vi "Framework Page.vi"(8 "error in (no error)":errorcluster, 11 "Node Ptr":T1 format="%.0x") -> (0 "error out":errorcluster)   [LabVIEW 2019, in "DSF System Explorer.lvlib"]
uses:
  DSF System Explorer.lvlib
  <vilib>/NI VeriStand/Custom Device API/Custom Device API.lvlib
  Shared/DSF Shared.lvlib
  <vilib>/NI VeriStand/Custom Device API/Custom Device Item Ref.ctl
panel:
  in  "SHDocVw.IWebBrowser":refnum<k7>(container)
  in  "New":bool
  in  "Configuration Version":string
  in  "Export":bool
  in  "Debug Mode":bool
  in  "Launch Data Viewer":bool
  in  "Server Frequency":dbl(ring)=20.0 items=["0.5 Hz"=0.5, "1.0 Hz"=1.0, "2.0 Hz"=2.0, "2.5 Hz"=2.5, "4.0 Hz"=4.0, "5.0 Hz"=5.0, "8.0 Hz"=8.0, "10.0 Hz"=10.0, "12.5 Hz"=12.5, "20.0 Hz"=20.0, "25.0 Hz"=25.0, "40.0 Hz"=40.0, "50.0 Hz"=50.0, "100.0 Hz"=100.0]
  in  "Enable Data Server":bool
  in  "Show Dialog on Error":bool
  in  "Show Threads":bool
  in  "Infinite FIFO Timeouts":bool
  in  "Measure Durations":bool
  in  "Measure Period":bool
  in  "Import":bool
  in  "View Configuration":bool
  # "Debug Options"
  # "Measurement Options"
  # "Data Server Options"
  # "All Targets"
  # "All Targets"
  # "All Targets"
  # "Windows Only"
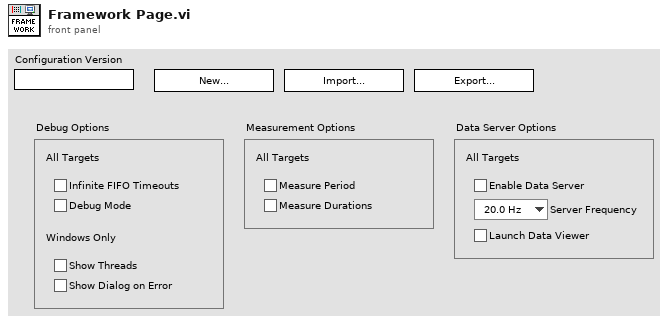
[diagram p1: front panel]
types:
  T1 = typedef "Custom Device API.lvlib/Custom Device Item Ref.ctl" = u64
  T2 = typedef "DSF Core.lvlibp/Framework.lvclass/Framework Options.ctl" = cluster{"FIFO Options":T3, "Thread Options":T4, "Plugin Options":T5, "Performance Options":T6, "Data Server Options":T7}
  T3 = typedef "DSF Core.lvlibp/Framework.lvclass/DSF FIFO Options.ctl" = cluster{"Infinite Timeouts":bool}
  T4 = typedef "DSF Core.lvlibp/Thread.lvclass/Thread Options.ctl" = cluster{"Show FP On Call":bool, "Close FP After Call":bool, "Allow Debugging":bool}
  T5 = typedef "DSF Core.lvlibp/Framework.lvclass/DSF Plugin Options.ctl" = cluster{"Default Components":bool}
  T6 = typedef "DSF Core.lvlibp/DSF Performance Options.ctl" = cluster{"Measure Period":bool, "Measure Rx/Tx Duration":bool}
  T7 = typedef "DSF Core.lvlibp/Framework.lvclass/Data Server Options.ctl" = cluster{"Enable Data Server":bool, "Period":u32}
  T8 = typedef "DSF Core.lvlibp/DSF Version Info.ctl" = cluster{"major":u32, "minor":u32, "fix":u32, "build":string}
  T9 = typedef "Custom Device API.lvlib/Custom Device Commands.ctl" = enum16{"Default", "Item renamed", "Shutdown", "Dynamic button pressed"}
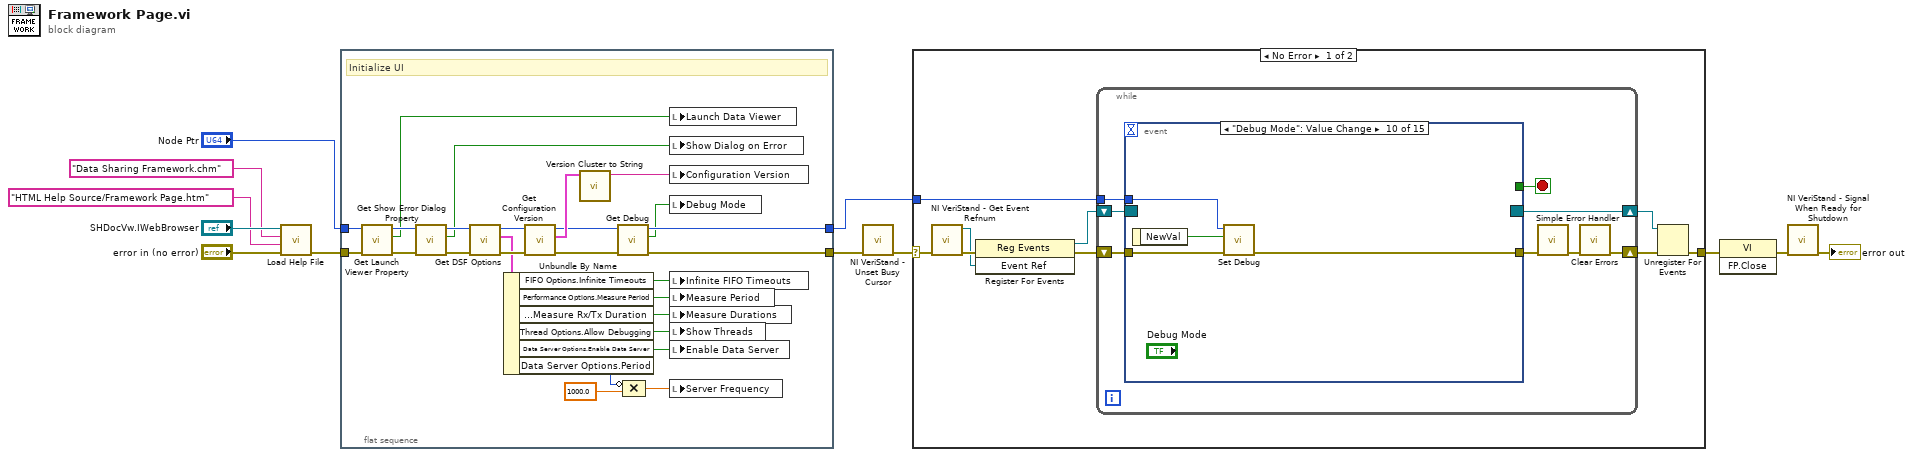
[diagram p0: block diagram]
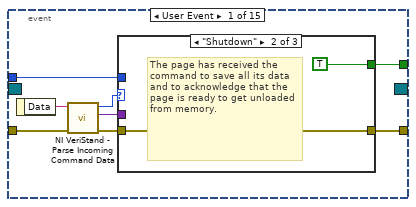
[diagram p2: hidden frame]
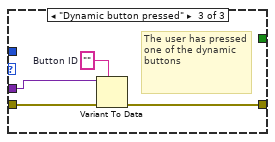
[diagram p4: hidden frame]
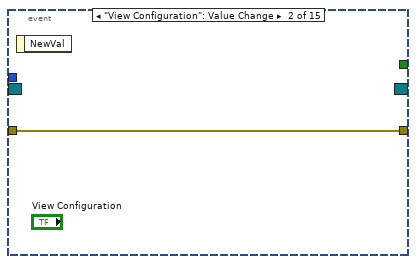
[diagram p5: hidden frame]
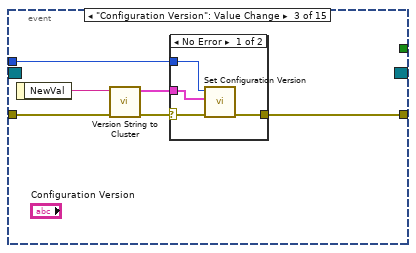
[diagram p6: hidden frame]
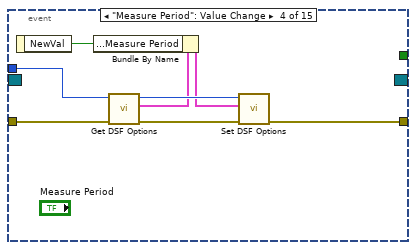
[diagram p8: hidden frame]
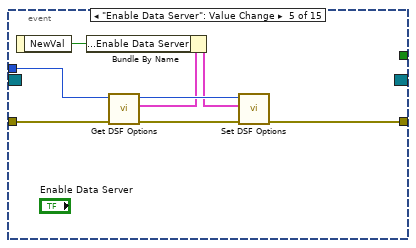
[diagram p9: hidden frame]
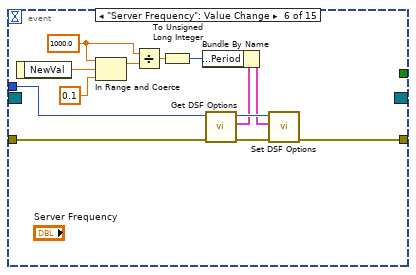
[diagram p10: hidden frame]
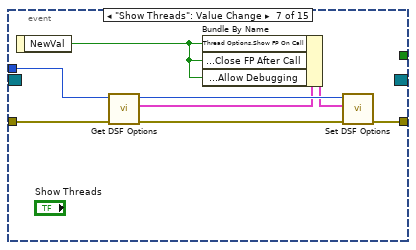
[diagram p11: hidden frame]
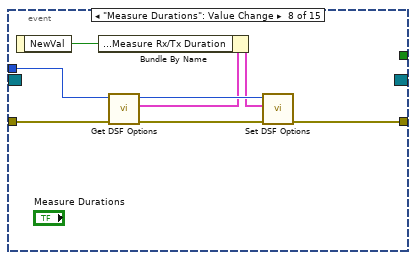
[diagram p12: hidden frame]
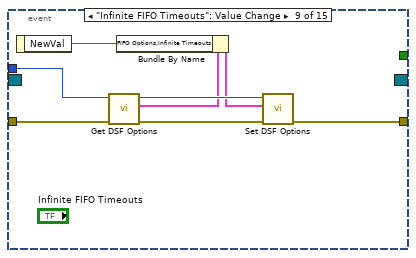
[diagram p13: hidden frame]
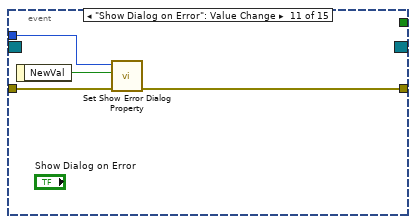
[diagram p14: hidden frame]
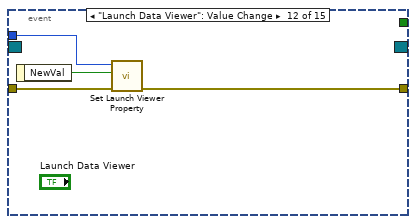
[diagram p15: hidden frame]
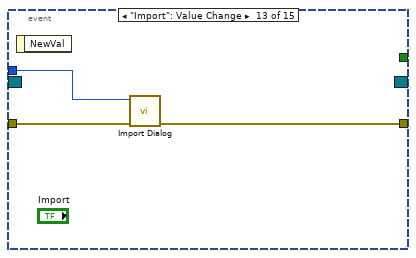
[diagram p16: hidden frame]
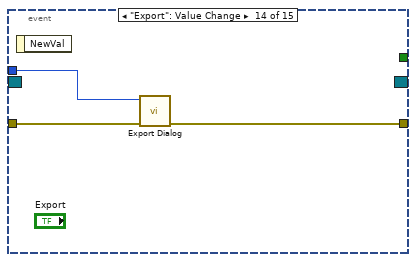
[diagram p17: hidden frame]
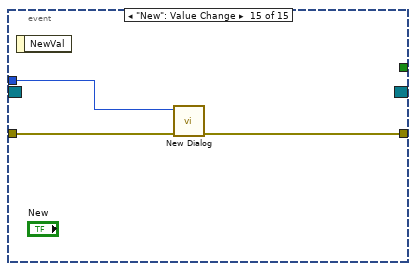
[diagram p18: hidden frame]
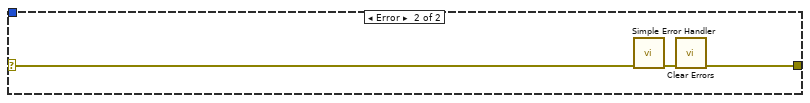
[diagram p19: hidden frame]
diagram:
  n1 = call "Load Help File.vi"("error in (no error)"="error in (no error)", "HTML File to Load"="HTML Help Source/Framework Page.htm" ("Main CHM File"), "Main CHM File"="Data Sharing Framework.chm", "Browser"="SHDocVw.IWebBrowser") -> ("error out"=w4:errorcluster)  [unwired: 7 in]
  n2 = flat-sequence "Initialization code" {
    tunnel: w4 -> [w28]
    tunnel: "Node Ptr" -> [w27]
    tunnel: [w14] -> w8
    tunnel: [w15] -> w6
    frame #0 {
      # "Initialize UI"
      n3 = call "Get Launch Viewer Property.vi"("error in (no error)"=w28, "Item Ref in"=w27) -> ("error out"=w26:errorcluster, "launch viewer"=w24:bool, "Item Ref out"=w25:T1)  [unwired: 7 in]
      n4 = call "Get Show Error Dialog Property.vi"("error in (no error)"=w26, "Item Ref in"=w25) -> ("error out"=w33:errorcluster, "show error dialog"=w29:bool, "Item Ref out"=w34:T1)  [unwired: 7 in]
      n5 = call "Get DSF Options.vi"("error in (no error)"=w33, "Item Ref in"=w34) -> ("error out"=w23:errorcluster, "options"=w21:T2, "Item Ref out"=w22:T1)  [unwired: 7 in]
      n6 = Unbundle By Name(w21) -> ("FIFO Options.Infinite Timeouts"=w38:bool, "Performance Options.Measure Period"=w37:bool, "Performance Options.Measure Rx/Tx Duration"=w36:bool, "Thread Options.Allow Debugging"=w35:bool, "Data Server Options.Enable Data Server"=w32:bool, "Data Server Options.Period"=w18:u32)
      n7 = call "Get Configuration Version.vi"("error in (no error)"=w23, "Item Ref in"=w22) -> ("error out"=w17:errorcluster, "version"=w20:T8, "Item Ref out"=w16:T1)  [unwired: 7 in]
      n8 = call "Version Cluster to String.vi"("version"=w20) -> ("version string"=w19:string)  [unwired: 9 in, 1 out]
      n9 = call "Get Debug.vi"("error in (no error)"=w17, "Item Ref in"=w16) -> ("error out"=w14:errorcluster, "debug"=w13:bool, "Item Ref out"=w15:T1)  [unwired: 7 in]
      n10 = Compound Arithmetic op=MULTIPLY(invert w18, 1000.0 ("y")) -> (w31:dbl)
      n11 = local write "Launch Data Viewer"(w24) -> ()
      n12 = local write "Show Dialog on Error"(w29) -> ()
      n13 = local write "Configuration Version"(w19) -> ()
      n14 = local write "Debug Mode"(w13) -> ()
      n15 = local write "Infinite FIFO Timeouts"(w38) -> ()
      n16 = local write "Measure Period"(w37) -> ()
      n17 = local write "Measure Durations"(w36) -> ()
      n18 = local write "Show Threads"(w35) -> ()
      n19 = local write "Enable Data Server"(w32) -> ()
      n20 = local write "Server Frequency"(w31) -> ()
    }
  }
  n21 = call <vilib>:"NI VeriStand - Unset Busy Cursor.vi"("error in (no error)"=w8) -> ("error out"=w7:errorcluster)  [unwired: 10 out]
  n22 = case shown="No Error" w7 {
    selector: w7 -> [w39 w159]
    tunnel: [w44 w157] -> w12
    tunnel: w6 -> [w40 _]
    frame No Error {
      n23 = call <vilib>:"NI VeriStand - Get Event Refnum.vi"("error in (no error)"=w39) -> ("error out"=w47:errorcluster, "Event Ref"=w43:refnum<user-event>)  [unwired: 9 out]
      n24 = register-events(error in=w47, w43) -> (reference out=w41:refnum<event-registration>, error out=w42:errorcluster)  [unwired: 1 in]
      n25 = while {
        tunnel: w40 -> [w51]
        shift-right: [w48] -> w45
        shift-left: w42 -> [w54]
        shift-right: [w55] -> w46
        shift-left: w41 -> [w53]
        stop <- w52 stop-if-true
        n26 = event shown="[9] \"Debug Mode\": Value Change" {
          selector: w53 -> [_ _ _ _ _ _ _ _ _ _ _ _ _ _ _]
          dyn-events: [_ _ _ _ _ _ _ _ _ _ _ _ _ _ _] -> w55
          timeout: _ -> [_ _ _ _ _ _ _ _ _ _ _ _ _ _ _]
          tunnel: w54 -> [w63 w71 w77 w88 w96 w110 w118 w125 w133 w139 w143 w147 w150 w153 w156]
          tunnel: [w59 _ _ _ _ _ _ _ _ _ _ _ _ _ _] -> w52
          tunnel: [w58 w71 w74 w85 w93 w108 w115 w122 w130 w136 w141 w146 w148 w151 w154] -> w50
          tunnel: w51 -> [w57 _ w72 w90 w98 w111 w119 w127 w135 w138 w142 w145 w149 w152 w155]
          event User Event {
            n27 = event-data() -> ("Data"=w62:string)  [unwired: 1 out]
            n28 = call <vilib>:"NI VeriStand - Parse Incoming Command Data.vi"("error in (no error)"=w63, "Incoming data"=w62) -> ("error out"=w61:errorcluster, "Outgoing data"=w56:variant, "Action"=w60:T9)  [unwired: 7 out]
            n29 = case shown="\"Shutdown\"" w60 {
              tunnel: w61 -> [w64 w65 w70]
              tunnel: [_ TRUE _] -> w59
              tunnel: [w64 w65 w67] -> w58
              tunnel: w57 -> [_ _ _]
              tunnel: w56 -> [_ _ w69]
              frame "Default", Default {
              }
              frame "Shutdown" {
                # "The page has received the command to save all its data and to acknowledge that the page is ready to get unloaded from memory."
              }
              frame "Dynamic button pressed" {
                w68 = ""  # Button ID
                # "The user has pressed one of the dynamic buttons"
                n30 = Variant To Data(error in=w70, type=w68, Variant=w69) -> (error out=w67:errorcluster)  [unwired: 1 out]
              }
            }
          }
          event "View Configuration": Value Change {
            n31 = event-data() -> ()  [unwired: 2 out]
          }
          event "Configuration Version": Value Change {
            n32 = event-data() -> ("NewVal"=w76:string)  [unwired: 1 out]
            n33 = call "Version String to Cluster.vi"("error in (no error)"=w77, "version string"=w76) -> ("error out"=w75:errorcluster, "version"=w73:T8)  [unwired: 8 in]
            n34 = case shown="No Error" w75 {
              selector: w75 -> [w81 w82]
              tunnel: [w78 w82] -> w74
              tunnel: w73 -> [w80 _]
              tunnel: w72 -> [w79 _]
              frame No Error {
                n35 = call "Set Configuration Version.vi"("error in (no error)"=w81, "version"=w80, "Item Ref in"=w79) -> ("error out"=w78:errorcluster)  [unwired: 7 in, 1 out]
              }
              frame Error {
              }
            }
          }
          event "Measure Period": Value Change {
            n36 = event-data() -> ("NewVal"=w89:bool)  [unwired: 1 out]
            n37 = call "Get DSF Options.vi"("error in (no error)"=w88, "Item Ref in"=w90) -> ("error out"=w86:errorcluster, "options"=w83:T2, "Item Ref out"=w87:T1)  [unwired: 7 in]
            n38 = Bundle By Name(cluster=w83, "Performance Options.Measure Period"=w89) -> (w84:T2)
            n39 = call "Set DSF Options.vi"("error in (no error)"=w86, "options"=w84, "Item Ref in"=w87) -> ("error out"=w85:errorcluster)  [unwired: 7 in, 1 out]
          }
          event "Enable Data Server": Value Change {
            n40 = event-data() -> ("NewVal"=w97:bool)  [unwired: 1 out]
            n41 = call "Get DSF Options.vi"("error in (no error)"=w96, "Item Ref in"=w98) -> ("error out"=w94:errorcluster, "options"=w91:T2, "Item Ref out"=w95:T1)  [unwired: 7 in]
            n42 = Bundle By Name(cluster=w91, "Data Server Options.Enable Data Server"=w97) -> (w92:T2)
            n43 = call "Set DSF Options.vi"("error in (no error)"=w94, "options"=w92, "Item Ref in"=w95) -> ("error out"=w93:errorcluster)  [unwired: 7 in, 1 out]
          }
          event "Server Frequency": Value Change {
            w101 = 1000.0 ("y")
            n44 = event-data() -> ("NewVal"=w103:dbl)  [unwired: 1 out]
            n45 = In Range and Coerce(upper limit=w101, x=w103, lower limit=0.1) -> (coerced(x)=w99:dbl)  [unwired: 1 out]
            n46 = Divide(x=w101, y=w99) -> (x/y=w100:dbl)
            n47 = To Unsigned Long Integer(number=w100) -> (unsigned 32bit integer=w105:u32)
            n48 = call "Get DSF Options.vi"("error in (no error)"=w110, "Item Ref in"=w111) -> ("error out"=w104:errorcluster, "options"=w106:T2, "Item Ref out"=w109:T1)  [unwired: 7 in]
            n49 = Bundle By Name(cluster=w106, "Data Server Options.Period"=w105) -> (w107:T2)
            n50 = call "Set DSF Options.vi"("error in (no error)"=w104, "options"=w107, "Item Ref in"=w109) -> ("error out"=w108:errorcluster)  [unwired: 7 in, 1 out]
          }
          event "Show Threads": Value Change {
            n51 = event-data() -> ("NewVal"=w112:bool)  [unwired: 1 out]
            n52 = call "Get DSF Options.vi"("error in (no error)"=w118, "Item Ref in"=w119) -> ("error out"=w116:errorcluster, "options"=w113:T2, "Item Ref out"=w117:T1)  [unwired: 7 in]
            n53 = Bundle By Name(cluster=w113, "Thread Options.Show FP On Call"=w112, "Thread Options.Close FP After Call"=w112, "Thread Options.Allow Debugging"=w112) -> (w114:T2)
            n54 = call "Set DSF Options.vi"("error in (no error)"=w116, "options"=w114, "Item Ref in"=w117) -> ("error out"=w115:errorcluster)  [unwired: 7 in, 1 out]
          }
          event "Measure Durations": Value Change {
            n55 = event-data() -> ("NewVal"=w126:bool)  [unwired: 1 out]
            n56 = call "Get DSF Options.vi"("error in (no error)"=w125, "Item Ref in"=w127) -> ("error out"=w123:errorcluster, "options"=w120:T2, "Item Ref out"=w124:T1)  [unwired: 7 in]
            n57 = Bundle By Name(cluster=w120, "Performance Options.Measure Rx/Tx Duration"=w126) -> (w121:T2)
            n58 = call "Set DSF Options.vi"("error in (no error)"=w123, "options"=w121, "Item Ref in"=w124) -> ("error out"=w122:errorcluster)  [unwired: 7 in, 1 out]
          }
          event "Infinite FIFO Timeouts": Value Change {
            n59 = event-data() -> ("NewVal"=w134:bool)  [unwired: 1 out]
            n60 = call "Get DSF Options.vi"("error in (no error)"=w133, "Item Ref in"=w135) -> ("error out"=w131:errorcluster, "options"=w128:T2, "Item Ref out"=w132:T1)  [unwired: 7 in]
            n61 = Bundle By Name(cluster=w128, "FIFO Options.Infinite Timeouts"=w134) -> (w129:T2)
            n62 = call "Set DSF Options.vi"("error in (no error)"=w131, "options"=w129, "Item Ref in"=w132) -> ("error out"=w130:errorcluster)  [unwired: 7 in, 1 out]
          }
          event "Debug Mode": Value Change {
            n63 = event-data() -> ("NewVal"=w137:bool)  [unwired: 1 out]
            n64 = call "Set Debug.vi"("error in (no error)"=w139, "debug"=w137, "Item Ref in"=w138) -> ("error out"=w136:errorcluster)  [unwired: 7 in, 1 out]
          }
          event "Show Dialog on Error": Value Change {
            n65 = event-data() -> ("NewVal"=w140:bool)  [unwired: 1 out]
            n66 = call "Set Show Error Dialog Property.vi"("error in (no error)"=w143, "show error dialog"=w140, "Item Ref in"=w142) -> ("error out"=w141:errorcluster)  [unwired: 7 in, 1 out]
          }
          event "Launch Data Viewer": Value Change {
            n67 = event-data() -> ("NewVal"=w144:bool)  [unwired: 1 out]
            n68 = call "Set Launch Viewer Property.vi"("error in (no error)"=w147, "launch viewer"=w144, "Item Ref in"=w145) -> ("error out"=w146:errorcluster)  [unwired: 7 in, 1 out]
          }
          event "Import": Value Change {
            n69 = event-data() -> ()  [unwired: 2 out]
            n70 = call "Import Dialog.vi"("error in"=w150, "Item Ref in"=w149) -> ("error out"=w148:errorcluster)  [unwired: 8 in, 1 out]
          }
          event "Export": Value Change {
            n71 = event-data() -> ()  [unwired: 2 out]
            n72 = call "Export Dialog.vi"("error in (no error)"=w153, "Item Ref in"=w152) -> ("error out"=w151:errorcluster)  [unwired: 8 in, 1 out]
          }
          event "New": Value Change {
            n73 = event-data() -> ()  [unwired: 2 out]
            n74 = call "New Dialog.vi"("error in (no error)"=w156, "Item Ref in"=w155) -> ("error out"=w154:errorcluster)  [unwired: 8 in, 1 out]
          }
        }
        n75 = call <vilib>:"Simple Error Handler.vi"("error in (no error)"=w50) -> ("error out"=w49:errorcluster)  [unwired: 1 in, 7 out]
        n76 = call <vilib>:"Clear Errors.vi"("error in (no error)"=w49) -> ("error out"=w48:errorcluster)  [unwired: 1 in, 5 out]
      }
      n77 = Unregister For Events(event registration refnum=w46, error in=w45) -> (error out=w44:errorcluster)
    }
    frame Error {
      n78 = call <vilib>:"Simple Error Handler.vi"("error in (no error)"=w159) -> ("error out"=w158:errorcluster)  [unwired: 1 in, 7 out]
      n79 = call <vilib>:"Clear Errors.vi"("error in (no error)"=w158) -> ("error out"=w157:errorcluster)  [unwired: 1 in, 5 out]
    }
  }
  n80 = invoke class="VI" method="FP.Close"(error in=w12) -> (error out=w11:errorcluster)  [unwired: 2 in, 2 out]
  n81 = call <vilib>:"NI VeriStand - Signal When Ready for Shutdown.vi"("error in (no error)"=w11) -> ("error out"=→"error out":errorcluster)  [unwired: 10 out]
